vi "Sample Up Down.vi"(7 "# Displayed Samples":i32=5, 8 "#  Available Samples":i32, 9 "Selected Sample in":i32, 10 "VKey":T1, 11 "Scrollbar Value in":i32) -> (2 "Selected Sample out":i32, 3 "Scrollbar Value out":i32)   [LabVIEW 2021]
uses:
  <vilib>/event_ctls.llb/eventvkey.ctl
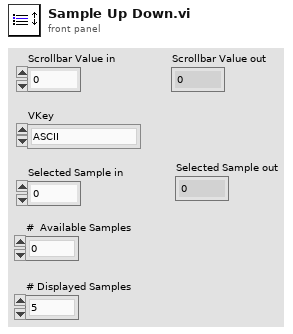
[diagram p1: front panel]
types:
  T1 = typedef "eventvkey.ctl" = enum16{"ASCII", "Enter", "Return", "Shift", "Ctrl", "Alt", "Cmd", "Opt", "Caps", "NumLock", "Clear", "Break", "Up", "Down", "Left", "Right", "Insert", "Delete", "Home", "End", "PageUp", "PageDown", "Escape", "Help", "Pause", "ScrollLock", "F1", "F2", "F3", "F4", "F5", "F6", "F7", "F8", "F9", "F10", "F11", "F12", "F13", "F14", "F15", "F16", "F17", "F18", "F19", "F20", "F21", "F22", "F23", "F24", "Play", "VolumeUp", "VolumeDown", "Mute", "Two Byte Char"}
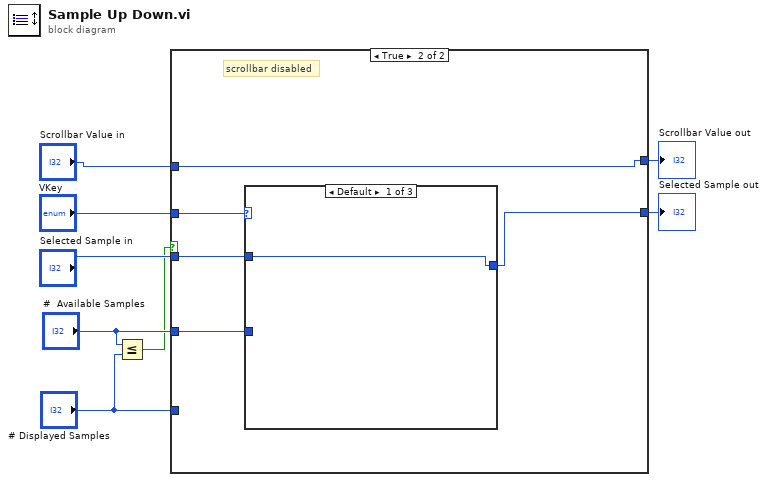
[diagram p0: block diagram]
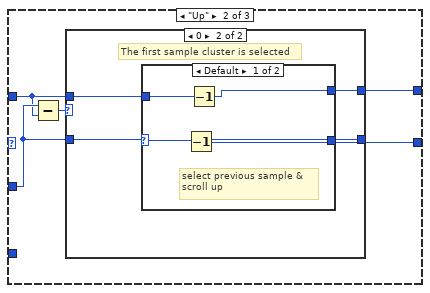
[diagram p3: hidden frame]
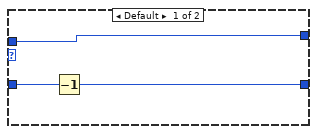
[diagram p4: hidden frame]
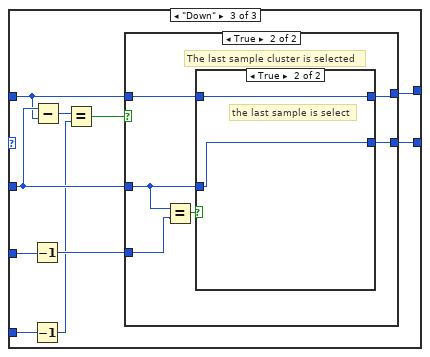
[diagram p6: hidden frame]
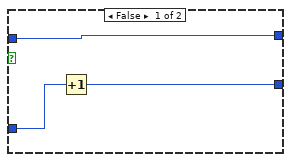
[diagram p7: hidden frame]
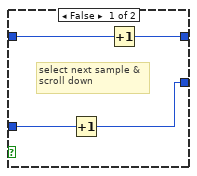
[diagram p8: hidden frame]
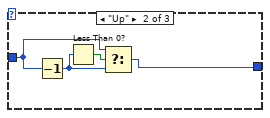
[diagram p9: hidden frame]
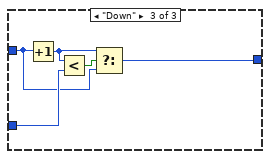
[diagram p10: hidden frame]
diagram:
  n1 = Less Or Equal?(x="#  Available Samples", y="# Displayed Samples") -> (x <= y?=w1:bool)
  n2 = case shown="True" w1 {
    tunnel: [w15 w65] -> w8
    tunnel: "Scrollbar Value in" -> [w14 w65]
    tunnel: [w13 w61] -> w6
    tunnel: "Selected Sample in" -> [w12 w63]
    tunnel: "VKey" -> [w11 w64]
    tunnel: "#  Available Samples" -> [w10 w62]
    tunnel: "# Displayed Samples" -> [w9 _]
    frame False {
      # "scrollbar enabled"
      n3 = case shown="Default" w11 {
        tunnel: w12 -> [w17 w19 w45]
        tunnel: [w17 w22 w42] -> w13
        tunnel: w14 -> [w16 w18 w44]
        tunnel: [w16 w21 w43] -> w15
        tunnel: w10 -> [_ _ w38]
        tunnel: w9 -> [_ _ w40]
        frame Default {
        }
        frame "Up" {
          n4 = Subtract(x=w19, y=w18) -> (x-y=w20:i32)
          n5 = case shown="0" w20 {
            tunnel: [w23 w26] -> w22
            tunnel: [w25 w27] -> w21
            tunnel: w19 -> [w24 w29]
            tunnel: w18 -> [w25 w28]
            frame Default {
              n6 = Decrement(x=w24) -> (x-1=w23:i32)
            }
            frame 0 {
              # "The first sample cluster is selected"
              n7 = case shown="Default" w29 {
                selector: w29 -> [w33 w34]
                tunnel: w28 -> [w31 w35]
                tunnel: [w30 w35] -> w27
                tunnel: [w32 w34] -> w26
                frame Default {
                  # "select previous sample & \nscroll up"
                  n8 = Decrement(x=w33) -> (x-1=w32:i32)
                  n9 = Decrement(x=w31) -> (x-1=w30:i32)
                }
                frame 0 {
                  # "the first sample is selected\n--> do nothing"
                }
              }
            }
          }
        }
        frame "Down" {
          n10 = Decrement(x=w38) -> (x-1=w37:i32)
          n11 = Decrement(x=w40) -> (x-1=w36:i32)
          n12 = Subtract(x=w45, y=w44) -> (x-y=w41:i32)
          n13 = Equal?(x=w41, y=w36) -> (x = y?=w39:bool)
          n14 = case shown="True" w39 {
            tunnel: [w46 w51] -> w42
            tunnel: [w48 w50] -> w43
            tunnel: w45 -> [w47 w53]
            tunnel: w44 -> [w48 w52]
            tunnel: w37 -> [_ w49]
            frame False {
              n15 = Increment(x=w47) -> (x+1=w46:i32)
            }
            frame True {
              # "The last sample cluster is selected"
              n16 = Equal?(x=w53, y=w49) -> (x = y?=w54:bool)
              n17 = case shown="True" w54 {
                tunnel: w53 -> [w56 w60]
                tunnel: w52 -> [w58 w59]
                tunnel: [w55 w60] -> w51
                tunnel: [w57 w59] -> w50
                frame False {
                  # "select next sample &\nscroll down"
                  n18 = Increment(x=w56) -> (x+1=w55:i32)
                  n19 = Increment(x=w58) -> (x+1=w57:i32)
                }
                frame True {
                  # "the last sample is select"
                }
              }
            }
          }
        }
      }
    }
    frame True {
      # "scrollbar disabled"
      n20 = case shown="Default" w64 {
        tunnel: w63 -> [w66 w68 w72]
        tunnel: w62 -> [_ _ w75]
        tunnel: [w66 w67 w71] -> w61
        frame Default {
        }
        frame "Up" {
          n21 = Decrement(x=w68) -> (x-1=w69:i32)
          n22 = Less Than 0?(x=w69) -> (x < 0?=w70:bool)
          n23 = Select(t=w68, s=w70, f=w69) -> (s? t:f=w67:i32)
        }
        frame "Down" {
          n24 = Increment(x=w72) -> (x+1=w73:i32)
          n25 = Less?(x=w73, y=w75) -> (x < y?=w74:bool)
          n26 = Select(t=w73, s=w74, f=w72) -> (s? t:f=w71:i32)
        }
      }
    }
  }
  "Scrollbar Value out" <- w8
  "Selected Sample out" <- w6
